vi "Conditional Menu Bar.vi"(0 "VI reference":refnum<vi>, 11 "error in (no error)":errorcluster) -> (15 "error out":errorcluster)   [LabVIEW 2015]
uses:
  <vilib>/Utility/config.llb/Read Key (Boolean).vi
  <vilib>/Utility/config.llb/NI_LVConfig.lvlib
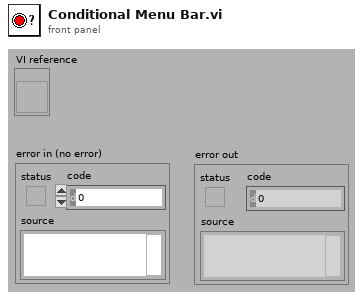
[diagram p1: front panel]
types:
  T1 = typedef "NI_LVConfig.lvlib/Config Data RefNum.ctl" = refnum<k1>
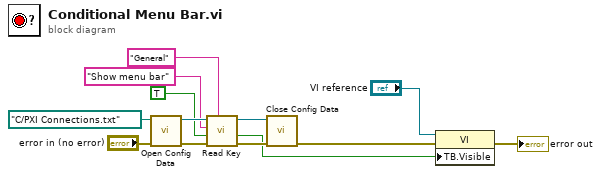
[diagram p0: block diagram]
diagram:
  n1 = call <vilib>:"Open Config Data.vi"("error in (no error)"="error in (no error)", "configuration file path"=path "C:/PXI Connections.txt") -> ("error out"=w9:errorcluster, "refnum"=w8:T1)  [unwired: 7 in, 1 out]
  n2 = call-poly <vilib>:"Read Key.vi"("section"="General", "error in (no error)"=w9, "default value"=TRUE, "key"="Show menu bar", "refnum"=w8) -> ("error out"=w4:errorcluster, "value"=w1:bool, "refnum out"=w3:T1)  [unwired: 3 in, 1 out]
  n3 = call <vilib>:"Close Config Data.vi"("error in (no error)"=w4, "refnum"=w3) -> ("error out"=w2:errorcluster)  [unwired: 8 in, 1 out]
  n4 = property class="VI"(reference="VI reference", error in=w2, "TB.Visible"=w1) -> (error out=→"error out":errorcluster)  [unwired: 1 out]
